vi "Set Power Parameters.vi"(8 "error in (no error)":errorcluster, 10 "Step In":refnum<k7>, 11 "Skyworks Spur Test in":refnum<class "Skyworks Spur Test.lvclass">) -> (0 "error out":errorcluster, 2 "Step Out":refnum<k7>, 3 "Skyworks Spur Test out":refnum<class "Skyworks Spur Test.lvclass">)   [LabVIEW 2018, in "Skyworks Spur Test.lvlib" / "Skyworks Spur Test.lvclass"]
uses:
  Skyworks Spur Test.lvclass
  Read SG Parameters.vi
  Read SA Parameters.vi
  Plugins/Measurement Interface.lvlibp/Measurement Interface.lvclass
  C:/Sequence Automation/Plugins/Measurement Interface.lvlibp/Measurement Interface.lvclass
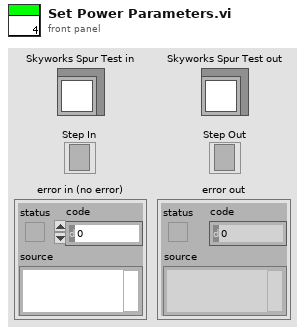
[diagram p1: front panel]
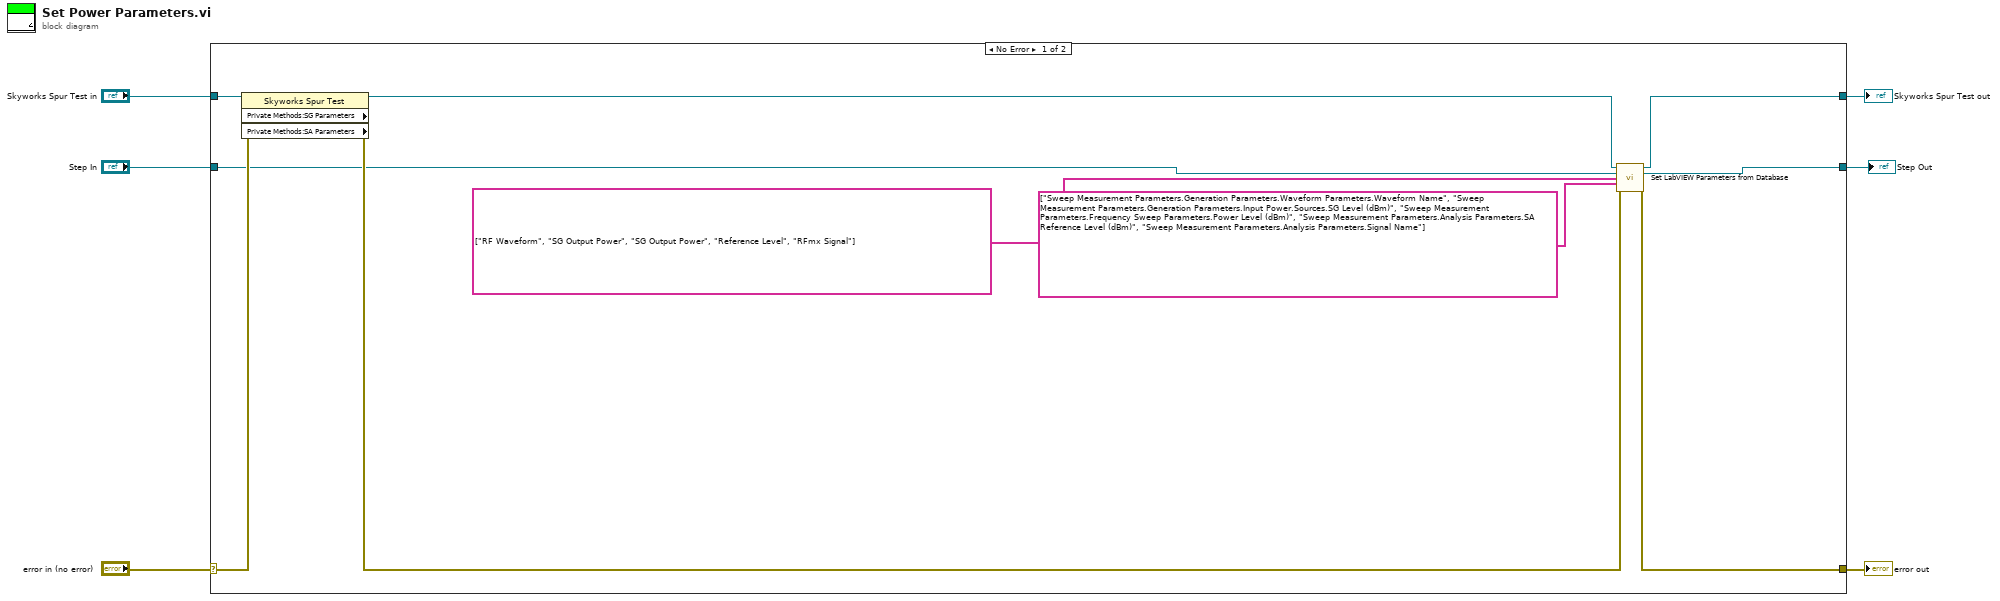
[diagram p0: block diagram]
diagram:
  n1 = case shown="No Error" "error in (no error)" {
    selector: "error in (no error)" -> [w16 w19]
    tunnel: [w13 w19] -> w5
    tunnel: [w9 w18] -> w3
    tunnel: "Skyworks Spur Test in" -> [w15 w18]
    tunnel: "Step In" -> [w12 w17]
    tunnel: [w11 w17] -> w1
    frame No Error {
      n2 = property class="Skyworks Spur Test" props=["Private Methods:SG Parameters", "Private Methods:SA Parameters"](reference=w15, error in=w16) -> (reference out=w10:refnum<class "Skyworks Spur Test.lvclass">, error out=w14:errorcluster)  [unwired: 2 out]
      n3 = call "Set LabVIEW Parameters from Database.vi"("Measurement Interface in"=w10, "Step In"=w12, "Dictionary Keys"=string[] ["RF Waveform", "SG Output Power", "SG Output Power", "Reference Level", "RFmx Signal"] ("Parameters to Set"), "LabVIEW Parameter Mapping"=string[] ["Sweep Measurement Parameters.Generation Parameters.Waveform Parameters.Waveform Name", "Sweep Measurement Parameters.Generation Parameters.Input Power.Sources.SG Level (dBm)", "Sweep Measurement Parameters.Frequency Sweep Parameters.Power Level (dBm)", "Sweep Measurement Parameters.Analysis Parameters.SA Reference Level (dBm)", "Sweep Measurement Parameters.Analysis Parameters.Signal Name"] ("Parameters to Set"), "error in (no error)"=w14) -> ("Measurement Interface out"=w9:refnum<class "Skyworks Spur Test.lvclass">, "Step Out"=w11:refnum<k7>, "error out"=w13:errorcluster)  [unwired: 8 in]
    }
    frame Error {
    }
  }
  "error out" <- w5
  "Skyworks Spur Test out" <- w3
  "Step Out" <- w1
